vi "Run_Point_Step.vi"(8 "error in (no error)":errorcluster, 9 "Producer In":T1, 10 "ScanQ In":refnum<queue>, 11 "SweepQ In":refnum<queue>) -> (0 "error out":errorcluster, 1 "Producer Out":T1, 2 "ScanQ Out":refnum<queue>, 3 "SweepQ Out":refnum<queue>)   [LabVIEW 2025]
uses:
  CTLS/Sweeper.ctl
  CTLS/Scan_Params (QMH).ctl
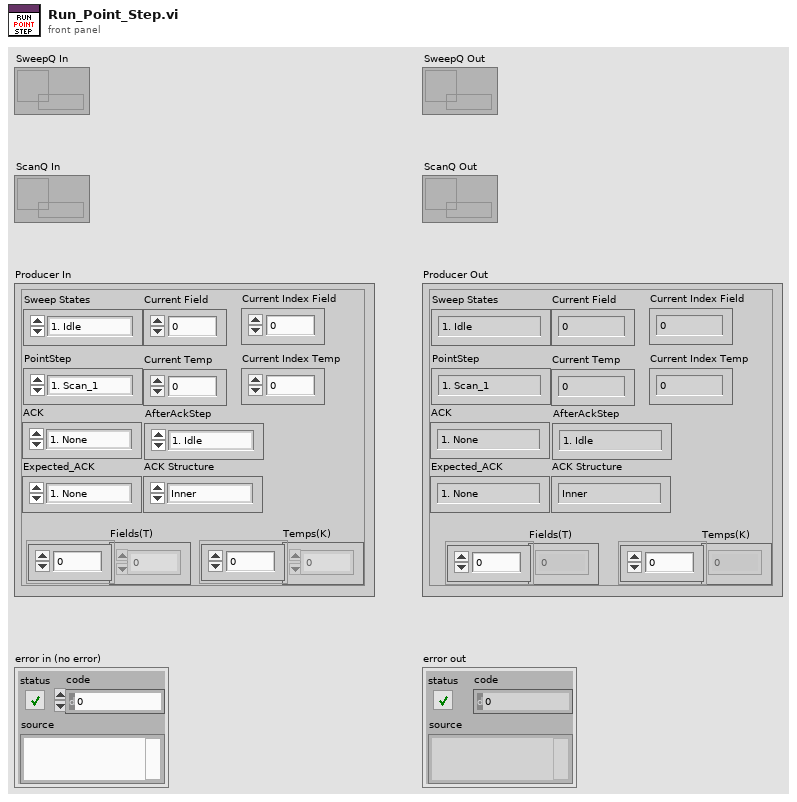
[diagram p1: front panel]
types:
  T1 = typedef "Sweeper.ctl" = cluster{"Temps(K)":dbl[], "Fields(T)":dbl[], "Sweep States":enum16{"1. Idle", "2. Start", "3. Apply_Config", "4. Run_Point_Step", "5. Wait ACK", "6. Next Field", "7. Next Temp", "8. Stop"}, "PointStep":enum16{"1. Scan_1", "2. DC_SF_1", "3. DC_BS_1", "4. Bias", "5. Scan_2", "6. DC_SF_2", "7. DC_BS_2", "8. Done"}, "Current Field":dbl, "Current Temp":dbl, "Expected_ACK":enum16{"1. None", "2. TempStable", "3. FieldStable", "4. ConfigApplied", "5. ScanDone", "6. BiasDone", "7. DriftDone (SF)", "8. DrifDone (BS)", "9. Done"}, "ACK":enum16{"1. None", "2. TempStable", "3. FieldStable", "4. ConfigApplied", "5. ScanDone", "6. BiasDone", "7. DriftDone (SF)", "8. DrifDone (BS)", "9. Done"}, "AfterAckStep":enum16{"1. Idle", "2. Start", "3. Apply_Config", "4. Run_Point_Step", "5. Wait ACK", "6. Next Field", "7. Next Temp", "8. Stop"}, "Current Index Field":i32, "Current Index Temp":i32, "ACK Structure ":enum16{"Inner", "Outer"}}
  T2 = enum16{"1. Scan_1", "2. DC_SF_1", "3. DC_BS_1", "4. Bias", "5. Scan_2", "6. DC_SF_2", "7. DC_BS_2", "8. Done"}
  T3 = enum16{"1. Idle", "2. Start", "3. Apply_Config", "4. Run_Point_Step", "5. Wait ACK", "6. Next Field", "7. Next Temp", "8. Stop"}
  T4 = enum16{"1. BIAS", "2. POLL BIAS", "3. SCAN", "4. SCAN_IDLE", "5. Drift_Correct (SF)", "6. Drift_Correct (BS)", "7. STOP"}
  T5 = enum16{"1. None", "2. TempStable", "3. FieldStable", "4. ConfigApplied", "5. ScanDone", "6. BiasDone", "7. DriftDone (SF)", "8. DrifDone (BS)", "9. Done"}
  T6 = typedef "Scan_Params (QMH).ctl" = cluster{"Setpoint (I)":dbl[], "Bias (V)":dbl[], "Number of scans":u8, "Port number (3364)":u32, "Avoid zero threshold (V)":dbl, "Current State":enum16{"1. BIAS", "2. POLL BIAS", "3. SCAN", "4. SCAN_IDLE", "5. Drift_Correct (SF)", "6. Drift_Correct (BS)", "7. STOP"}}
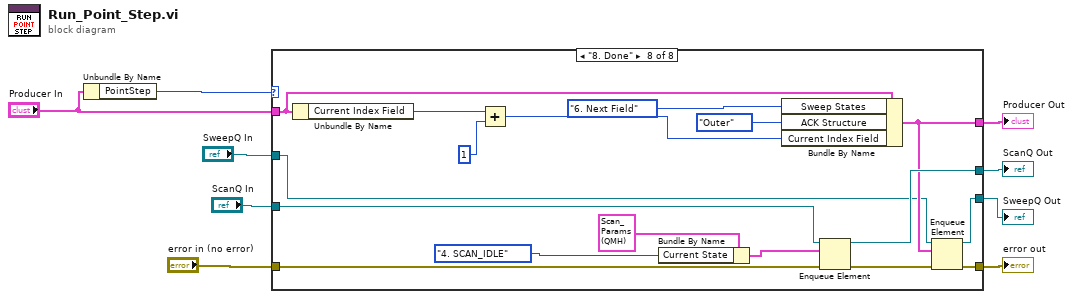
[diagram p0: block diagram]
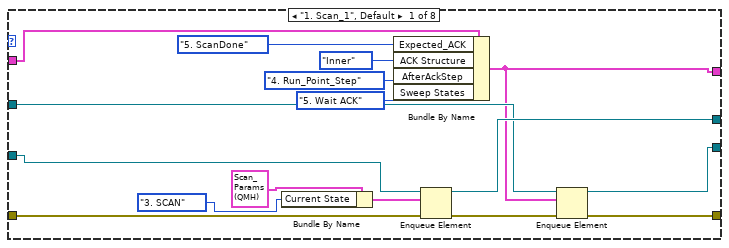
[diagram p2: hidden frame]
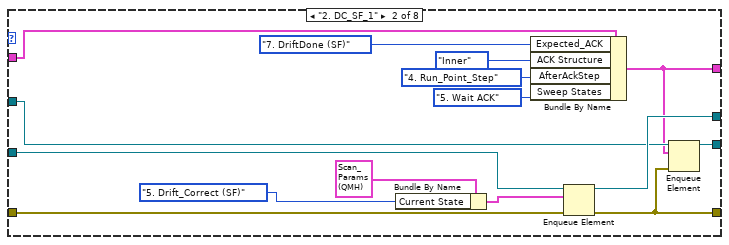
[diagram p3: hidden frame]
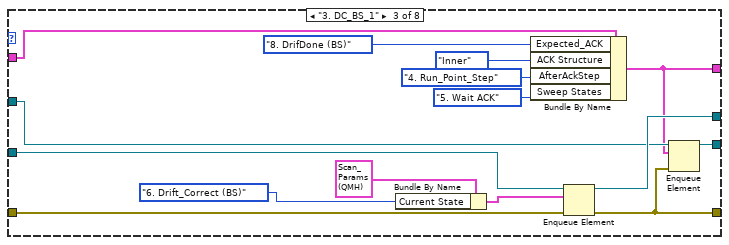
[diagram p4: hidden frame]
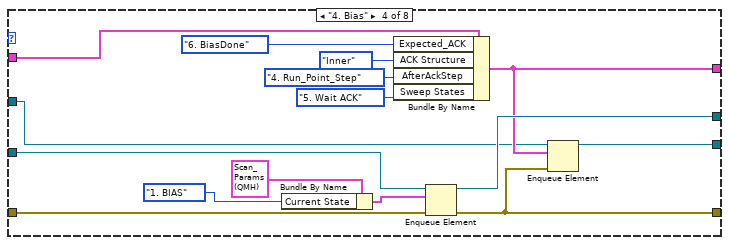
[diagram p5: hidden frame]
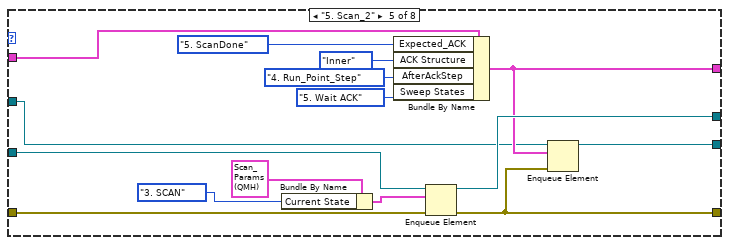
[diagram p6: hidden frame]
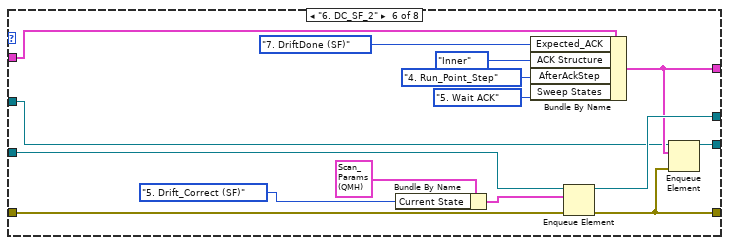
[diagram p7: hidden frame]
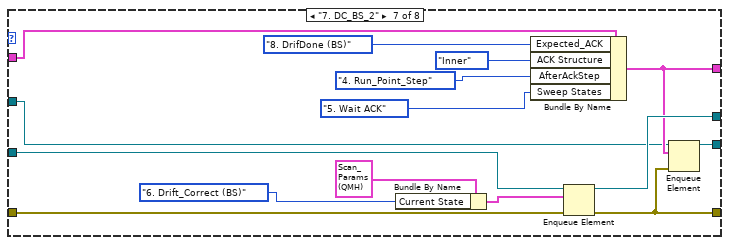
[diagram p8: hidden frame]
diagram:
  n1 = Unbundle By Name("Producer In") -> ("PointStep"=w5:T2)
  n2 = case shown="\"8. Done\"" w5 {
    tunnel: "ScanQ In" -> [w25 w34 w48 w64 w79 w94 w109 w127]
    tunnel: "Producer In" -> [w22 w31 w50 w65 w77 w95 w110 w120]
    tunnel: [w14 w29 w44 w61 w76 w91 w106 w126] -> w8
    tunnel: "error in (no error)" -> [w19 w35 w47 w63 w78 w93 w108 w128]
    tunnel: [w18 w36 w49 w62 w80 w92 w107 w129] -> w4
    tunnel: [w16 w32 w46 w59 w74 w89 w105 w124] -> w3
    tunnel: "SweepQ In" -> [w15 w30 w45 w60 w75 w90 w104 w125]
    tunnel: [w12 w28 w43 w58 w73 w88 w103 w122] -> w1
    frame "1. Scan_1", Default {
      n3 = Bundle By Name(cluster=T6 {"Setpoint (I)"=[], "Bias (V)"=[], "Number of scans"=1, "Port number (3364)"=3364, "Avoid zero threshold (V)"=0.004999999888241291, "Current State"=enum."1. BIAS"} ("Scan Parameters"), "Current State"=T4."3. SCAN") -> (w23:T6)
      n4 = Bundle By Name(cluster=w22, "Expected_ACK"=T5."5. ScanDone", "ACK Structure"=enum16{"Inner", "Outer"}."Inner", "AfterAckStep"=T3."4. Run_Point_Step", "Sweep States"=T3."5. Wait ACK") -> (w14:T1)
      n5 = Enqueue Element(queue=w25, element=w23, error in (no error)=w19) -> (queue out=w18:refnum<queue>, error out=w13:errorcluster)  [unwired: 1 in, 1 out]
      n6 = Enqueue Element(queue=w15, element=w14, error in (no error)=w13) -> (queue out=w16:refnum<queue>, error out=w12:errorcluster)  [unwired: 1 in, 1 out]
    }
    frame "2. DC_SF_1" {
      n7 = Bundle By Name(cluster=T6 {"Setpoint (I)"=[], "Bias (V)"=[], "Number of scans"=1, "Port number (3364)"=3364, "Avoid zero threshold (V)"=0.004999999888241291, "Current State"=enum."1. BIAS"} ("Scan Parameters"), "Current State"=T4."5. Drift_Correct (SF)") -> (w39:T6)
      n8 = Bundle By Name(cluster=w31, "Expected_ACK"=T5."7. DriftDone (SF)", "ACK Structure"=enum16{"Inner", "Outer"}."Inner", "AfterAckStep"=T3."4. Run_Point_Step", "Sweep States"=T3."5. Wait ACK") -> (w29:T1)
      n9 = Enqueue Element(queue=w34, element=w39, error in (no error)=w35) -> (queue out=w36:refnum<queue>, error out=w28:errorcluster)  [unwired: 1 in, 1 out]
      n10 = Enqueue Element(queue=w30, element=w29, error in (no error)=w28) -> (queue out=w32:refnum<queue>)  [unwired: 1 in, 2 out]
    }
    frame "3. DC_BS_1" {
      n11 = Bundle By Name(cluster=T6 {"Setpoint (I)"=[], "Bias (V)"=[], "Number of scans"=1, "Port number (3364)"=3364, "Avoid zero threshold (V)"=0.004999999888241291, "Current State"=enum."1. BIAS"} ("Scan Parameters"), "Current State"=T4."6. Drift_Correct (BS)") -> (w54:T6)
      n12 = Bundle By Name(cluster=w50, "Expected_ACK"=T5."8. DrifDone (BS)", "ACK Structure"=enum16{"Inner", "Outer"}."Inner", "AfterAckStep"=T3."4. Run_Point_Step", "Sweep States"=T3."5. Wait ACK") -> (w44:T1)
      n13 = Enqueue Element(queue=w48, element=w54, error in (no error)=w47) -> (queue out=w49:refnum<queue>, error out=w43:errorcluster)  [unwired: 1 in, 1 out]
      n14 = Enqueue Element(queue=w45, element=w44, error in (no error)=w43) -> (queue out=w46:refnum<queue>)  [unwired: 1 in, 2 out]
    }
    frame "4. Bias" {
      n15 = Bundle By Name(cluster=T6 {"Setpoint (I)"=[], "Bias (V)"=[], "Number of scans"=1, "Port number (3364)"=3364, "Avoid zero threshold (V)"=0.004999999888241291, "Current State"=enum."1. BIAS"} ("Scan Parameters"), "Current State"=T4."1. BIAS") -> (w69:T6)
      n16 = Bundle By Name(cluster=w65, "Expected_ACK"=T5."6. BiasDone", "ACK Structure"=enum16{"Inner", "Outer"}."Inner", "AfterAckStep"=T3."4. Run_Point_Step", "Sweep States"=T3."5. Wait ACK") -> (w61:T1)
      n17 = Enqueue Element(queue=w64, element=w69, error in (no error)=w63) -> (queue out=w62:refnum<queue>, error out=w58:errorcluster)  [unwired: 1 in, 1 out]
      n18 = Enqueue Element(queue=w60, element=w61, error in (no error)=w58) -> (queue out=w59:refnum<queue>)  [unwired: 1 in, 2 out]
    }
    frame "5. Scan_2" {
      n19 = Bundle By Name(cluster=T6 {"Setpoint (I)"=[], "Bias (V)"=[], "Number of scans"=1, "Port number (3364)"=3364, "Avoid zero threshold (V)"=0.004999999888241291, "Current State"=enum."1. BIAS"} ("Scan Parameters"), "Current State"=T4."3. SCAN") -> (w84:T6)
      n20 = Bundle By Name(cluster=w77, "Expected_ACK"=T5."5. ScanDone", "ACK Structure"=enum16{"Inner", "Outer"}."Inner", "AfterAckStep"=T3."4. Run_Point_Step", "Sweep States"=T3."5. Wait ACK") -> (w76:T1)
      n21 = Enqueue Element(queue=w79, element=w84, error in (no error)=w78) -> (queue out=w80:refnum<queue>, error out=w73:errorcluster)  [unwired: 1 in, 1 out]
      n22 = Enqueue Element(queue=w75, element=w76, error in (no error)=w73) -> (queue out=w74:refnum<queue>)  [unwired: 1 in, 2 out]
    }
    frame "6. DC_SF_2" {
      n23 = Bundle By Name(cluster=T6 {"Setpoint (I)"=[], "Bias (V)"=[], "Number of scans"=1, "Port number (3364)"=3364, "Avoid zero threshold (V)"=0.004999999888241291, "Current State"=enum."1. BIAS"} ("Scan Parameters"), "Current State"=T4."5. Drift_Correct (SF)") -> (w99:T6)
      n24 = Bundle By Name(cluster=w95, "Expected_ACK"=T5."7. DriftDone (SF)", "ACK Structure"=enum16{"Inner", "Outer"}."Inner", "AfterAckStep"=T3."4. Run_Point_Step", "Sweep States"=T3."5. Wait ACK") -> (w91:T1)
      n25 = Enqueue Element(queue=w94, element=w99, error in (no error)=w93) -> (queue out=w92:refnum<queue>, error out=w88:errorcluster)  [unwired: 1 in, 1 out]
      n26 = Enqueue Element(queue=w90, element=w91, error in (no error)=w88) -> (queue out=w89:refnum<queue>)  [unwired: 1 in, 2 out]
    }
    frame "7. DC_BS_2" {
      n27 = Bundle By Name(cluster=T6 {"Setpoint (I)"=[], "Bias (V)"=[], "Number of scans"=1, "Port number (3364)"=3364, "Avoid zero threshold (V)"=0.004999999888241291, "Current State"=enum."1. BIAS"} ("Scan Parameters"), "Current State"=T4."6. Drift_Correct (BS)") -> (w114:T6)
      n28 = Bundle By Name(cluster=w110, "Expected_ACK"=T5."8. DrifDone (BS)", "ACK Structure"=enum16{"Inner", "Outer"}."Inner", "AfterAckStep"=T3."4. Run_Point_Step" ("Sweep States"), "Sweep States"=T3."5. Wait ACK" ("AfterAckStep")) -> (w106:T1)
      n29 = Enqueue Element(queue=w109, element=w114, error in (no error)=w108) -> (queue out=w107:refnum<queue>, error out=w103:errorcluster)  [unwired: 1 in, 1 out]
      n30 = Enqueue Element(queue=w104, element=w106, error in (no error)=w103) -> (queue out=w105:refnum<queue>)  [unwired: 1 in, 2 out]
    }
    frame "8. Done" {
      n31 = Unbundle By Name(w120) -> ("Current Index Field"=w116:i32)
      n32 = Add(x=w116, y=1) -> (x+y=w119:i32)
      n33 = Bundle By Name(cluster=T6 {"Setpoint (I)"=[], "Bias (V)"=[], "Number of scans"=1, "Port number (3364)"=3364, "Avoid zero threshold (V)"=0.004999999888241291, "Current State"=enum."1. BIAS"} ("Scan Parameters"), "Current State"=T4."4. SCAN_IDLE") -> (w131:T6)
      n34 = Bundle By Name(cluster=w120, "Sweep States"=T3."6. Next Field", "ACK Structure"=enum16{"Inner", "Outer"}."Outer", "Current Index Field"=w119) -> (w126:T1)
      n35 = Enqueue Element(queue=w127, element=w131, error in (no error)=w128) -> (queue out=w129:refnum<queue>, error out=w123:errorcluster)  [unwired: 1 in, 1 out]
      n36 = Enqueue Element(queue=w125, element=w126, error in (no error)=w123) -> (queue out=w124:refnum<queue>, error out=w122:errorcluster)  [unwired: 1 in, 1 out]
    }
  }
  "error out" <- w1
  "Producer Out" <- w8
  "ScanQ Out" <- w4
  "SweepQ Out" <- w3
